vi "Draw Scale Line.vi"(4 "draw area cache":T1, 5 "font size":i16, 6 "scale color":u32(colorbox)=16448250, 7 "scale label":string, 9 "line size (0-1)":dbl=0.05, 10 "heading (rad)":dbl, 11 "picture in":picture) -> (3 "picture out":picture)   [LabVIEW 2017, in "NI_Robotics_Compass Picture.lvlib"]
uses:
  <vilib>/robotics/Controls/Compass Indicator/Compass Picture/NI_Robotics_Compass Picture.lvlib
  <vilib>/robotics/Controls/Compass Indicator/Compass Picture/Draw Area State.ctl
  <vilib>/Utility/miscctls.llb/LVBoundsTypeDef.ctl
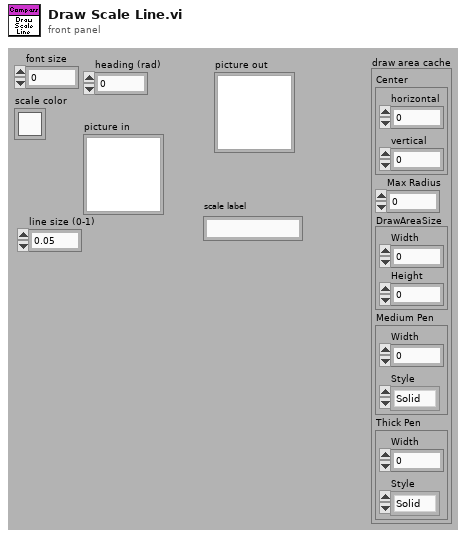
[diagram p1: front panel]
types:
  T1 = typedef "NI_Robotics_Compass Picture.lvlib/Draw Area State.ctl" = cluster{"Center":cluster{"horizontal":i16, "vertical":i16}, "Max Radius":dbl, "DrawAreaSize":T2, "Medium Pen":cluster{"Width":u16, "Style":enum32{"Solid", "Dash", "Dot", "DashDot", "DashDotDot"}}, "Thick Pen":cluster{"Width":u16, "Style":enum32{"Solid", "Dash", "Dot", "DashDot", "DashDotDot"}}}
  T2 = typedef "LVBoundsTypeDef.ctl" = cluster{"Width":u32, "Height":u32}
  T3 = enum16{"User-specified Font", "Application Font", "System Font", "Dialog Font"}
  T4 = cluster{"Font Name:":string, "Size":i16, "Strikeout?":bool, "Italic?":bool, "Underline?":bool, "Outline?":bool, "Shadow?":bool, "Bold?":bool}
  T5 = cluster{"horizontal":enum16{"left", "center", "right"}, "vertical":enum16{"top", "center", "bottom"}}
  T6 = cluster{"Width":u16, "Style":enum32{"Solid", "Dash", "Dot", "DashDot", "DashDotDot"}}
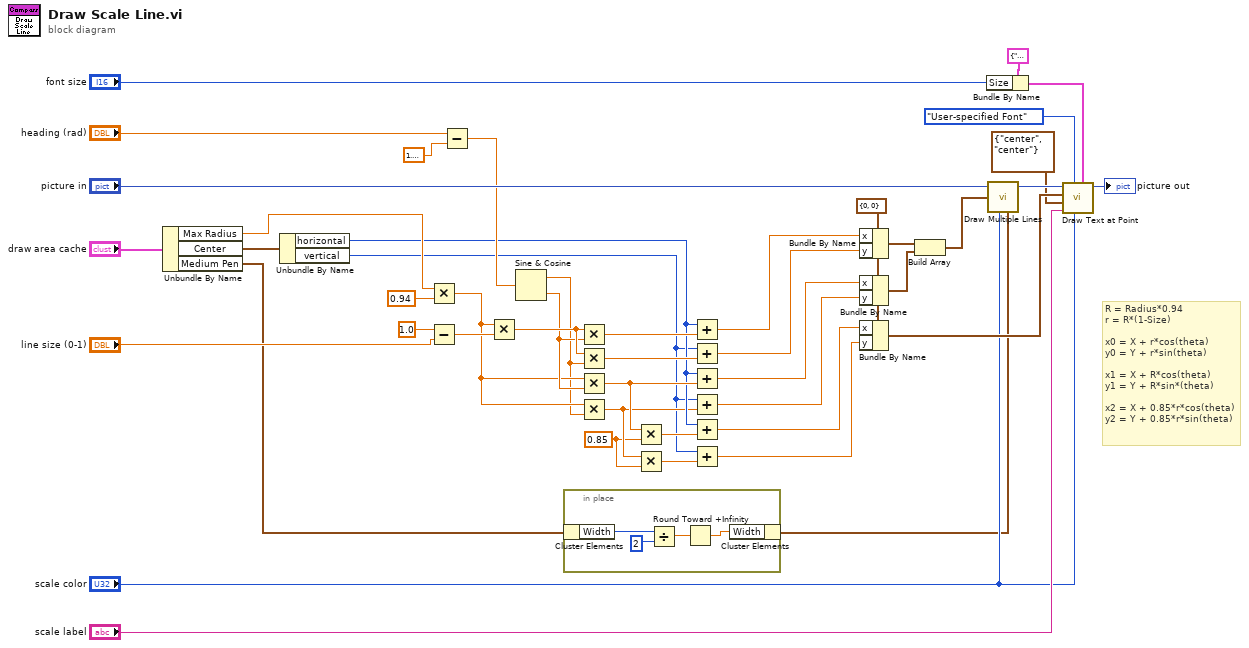
[diagram p0: block diagram]
diagram:
  w6 = 0.85 ("y")
  w39 = cluster{"x":i16, "y":i16} {"x"=0, "y"=0}
  # "R = Radius*0.94\nr = R*(1-Size)\n\nx0 = X + r*cos(theta)\ny0 = Y + r*sin(theta)\n\nx1 = X + R*cos(theta)\ny1 = Y + R*sin*(theta)\n\nx2 = X + 0.85*r*cos(theta)\ny2 = Y + 0.85*r*sin(theta)"
  n1 = Unbundle By Name("draw area cache") -> ("Max Radius"=w27:dbl, "Center"=w30:cluster{"horizontal":i16, "vertical":i16}, "Medium Pen"=w1:T6)
  n2 = Unbundle By Name(w30) -> ("horizontal"=w9:i16, "vertical"=w4:i16)
  n3 = Multiply(x=w27, y=0.94) -> (x*y=w14:dbl)
  n4 = Subtract(x=1.0, y="line size (0-1)") -> (x-y=w23:dbl)
  n5 = Subtract(x="heading (rad)", y=1.5707963267948966) -> (x-y=w22:dbl)
  n6 = Multiply(x=w14, y=w23) -> (x*y=w19:dbl)
  n7 = Sine & Cosine(0:w22) -> (1:w13:dbl, 2:w16:dbl)
  n8 = in-place {
    n9 = in-place-cluster #1(w1) -> ("Width"=w49:u16)
    n10 = Divide(x=w49, y=u16 2) -> (x/y=w48:dbl)
    n11 = Round Toward +Infinity(x=w48) -> (ceil(x): smallest int >= x=w47:dbl)
    n12 = in-place-cluster #1("Width"=w47) -> (w2:T6)
  }
  n13 = Multiply(x=w19, y=w16) -> (x*y=w21:dbl)
  n14 = Multiply(x=w19, y=w13) -> (x*y=w18:dbl)
  n15 = Multiply(x=w14, y=w16) -> (x*y=w11:dbl)
  n16 = Multiply(x=w14, y=w13) -> (x*y=w7:dbl)
  n17 = Multiply(x=w11, y=w6) -> (x*y=w10:dbl)
  n18 = Multiply(x=w7, y=w6) -> (x*y=w5:dbl)
  n19 = Add(x=w9, y=w21) -> (x+y=w20:dbl)
  n20 = Add(x=w4, y=w18) -> (x+y=w17:dbl)
  n21 = Add(x=w9, y=w11) -> (x+y=w15:dbl)
  n22 = Add(x=w4, y=w7) -> (x+y=w12:dbl)
  n23 = Add(x=w9, y=w10) -> (x+y=w8:dbl)
  n24 = Add(x=w4, y=w5) -> (x+y=w3:dbl)
  n25 = Bundle By Name(cluster=w39, "x"=w20, "y"=w17) -> (w44:cluster{"x":i16, "y":i16})
  n26 = Bundle By Name(cluster=w39, "x"=w15, "y"=w12) -> (w45:cluster{"x":i16, "y":i16})
  n27 = Bundle By Name(cluster=w39, "x"=w8, "y"=w3) -> (w38:cluster{"x":i16, "y":i16})
  n28 = Build Array(w44, w45) -> (w46:cluster{"x":i16, "y":i16}[])
  n29 = Bundle By Name(cluster=T4 {"Font Name:"="Calibri", "Size"=14, "Strikeout?"=FALSE, "Italic?"=FALSE, "Underline?"=FALSE, "Outline?"=FALSE, "Shadow?"=FALSE, "Bold?"=TRUE} ("[user-specified font]"), "Size"="font size") -> (w32:T4)
  n30 = call <vilib>:"Draw Multiple Lines.vi"("picture"="picture in", "line endpoints"=w46, "color(black)"="scale color", "pen"=w2) -> ("new picture"=w41:picture)  [unwired: 5 in]
  n31 = call <vilib>:"Draw Text at Point.vi"("[user-specified font]"=w32, "text color(black)"="scale color", "desired font(Application)"=T3."User-specified Font", "text"="scale label", "alignment(left, top)"=T5 {"horizontal"=enum."center", "vertical"=enum."center"}, "origin"=w38, "picture"=w41) -> ("new picture"=→"picture out":picture)  [unwired: 3 in, 1 out]
